vi "Configure FFT Display.vi"(8 "error in (no error)":errorcluster, 10 "FFT Display Mode (0: Normal)":i32(ring) items=["Normal", "Average", "Max Hold", "Min Hold"], 11 "VISA resource name":refnum<visa-resource-name>) -> (0 "error out":errorcluster, 3 "VISA resource name out":refnum<visa-resource-name>)   [LabVIEW 2015, in "Agilent 2000 3000 X-Series.lvlib"]
doc: "Sets the display mode for the FFT function.\n\nNotes:\nOnly applicable for 3000 T, 3000G, Series. \nThe FFT subsystem controls the FFT function in the oscilloscope."
uses:
  Agilent 2000 3000 X-Series.lvlib
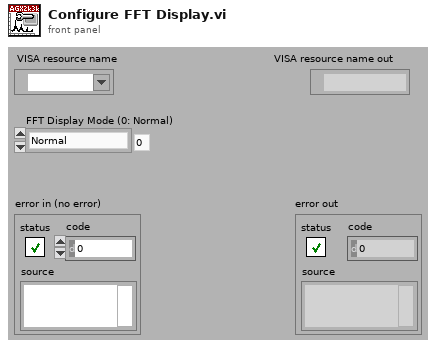
[diagram p1: front panel]
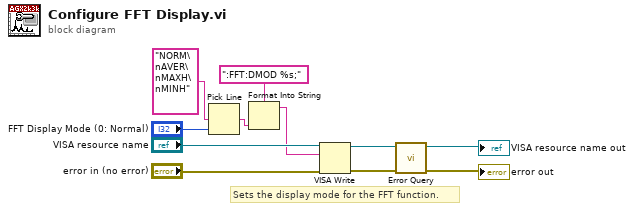
[diagram p0: block diagram]
diagram:
  # "Sets the display mode for the FFT function."
  n1 = Pick Line(multi-line string="NORM\nAVER\nMAXH\nMINH", line index="FFT Display Mode (0: Normal)") -> (output string=w2:string)  [unwired: 1 in]
  n2 = Format Into String(format string=":FFT:DMOD %s;", w2) -> (resulting string=w6:string)  [unwired: 2 in, 1 out]
  n3 = VISA Write(VISA resource name="VISA resource name", write buffer=w6, error in (no error)="error in (no error)") -> (VISA resource name out=w10:refnum<visa-resource-name>, error out=w9:errorcluster)  [unwired: 1 out]
  n4 = call "Error Query.vi"("error in (no error)"=w9, "VISA resource name"=w10) -> ("error out"=→"error out":errorcluster, "VISA resource name out"=→"VISA resource name out":refnum<visa-resource-name>)  [unwired: 8 out]
